vi "Initialize Trigger (SubVI).vi"() -> (3 "Refnum out":refnum<k21>)   [LabVIEW 2015]
uses:
  <vilib>/Utility/config.llb/Read Key (String).vi
  <vilib>/DAQmx/create/channels.llb/DAQmx Create Channel (DO-Digital Output).vi
  <vilib>/Utility/config.llb/NI_LVConfig.lvlib
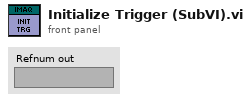
[diagram p1: front panel]
types:
  T1 = typedef "NI_LVConfig.lvlib/Config Data RefNum.ctl" = refnum<k1>
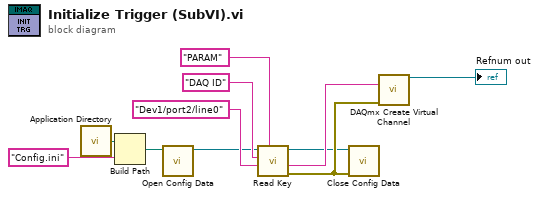
[diagram p0: block diagram]
diagram:
  n1 = call <vilib>:"Application Directory.vi"() -> ("Application Directory"=w9:path)
  n2 = Build Path(base path=w9, name or relative path="Config.ini") -> (appended path=w5:path)
  n3 = call <vilib>:"Open Config Data.vi"("configuration file path"=w5) -> ("refnum"=w1:T1)  [unwired: 8 in, 2 out]
  n4 = call-poly <vilib>:"Read Key.vi"("section"="PARAM", "default value"="Dev1/port2/line0", "key"="DAQ ID", "refnum"=w1) -> ("error out"=w8:errorcluster, "value"=w7:string, "refnum out"=w4:T1)  [unwired: 4 in, 1 out]
  n5 = call <vilib>:"Close Config Data.vi"("error in (no error)"=w8, "refnum"=w4) -> ()  [unwired: 8 in, 2 out]
  n6 = call-poly <vilib>:"DAQmx Create Virtual Channel.vi"("lines"=w7, "error in"=w8) -> ("task out"=→"Refnum out":refnum<k21>)  [unwired: 12 in, 1 out]
